vi "Average_array.vi"(1 "Input Array":dbl[](array[numeric]), 2 "Average over..":dbl) -> (0 "Output Array":dbl[](array[numeric]))   [LabVIEW 2016]
panel:
  out "Waveform Graph":dbl[](graph)
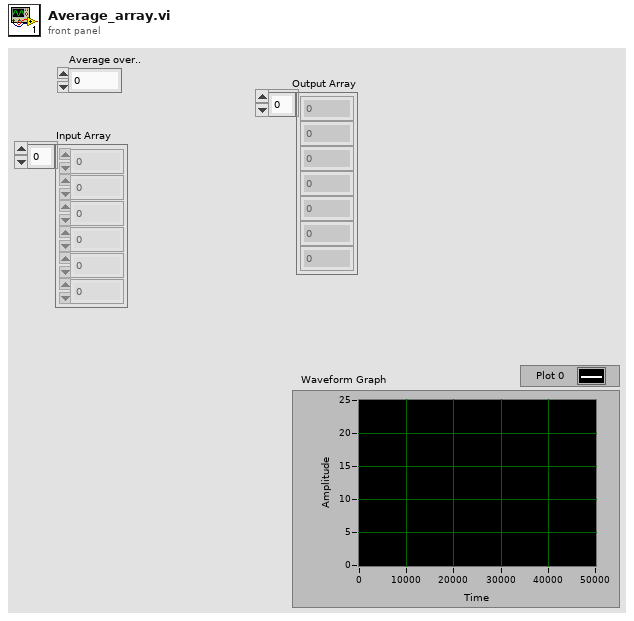
[diagram p1: front panel]
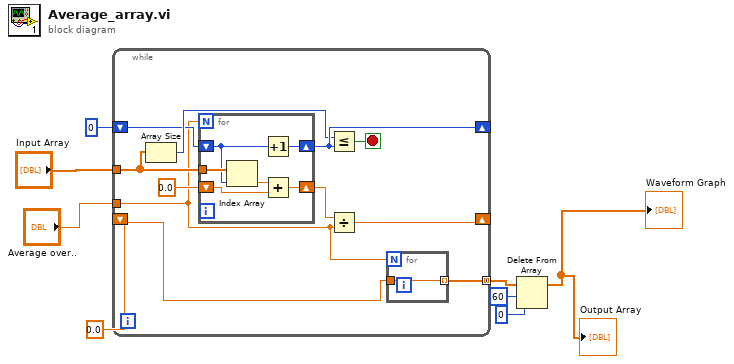
[diagram p0: block diagram]
diagram:
  n1 = while {
    tunnel: "Average over.." -> [w10]
    tunnel: "Input Array" -> [w16]
    shift-right: [w15] -> _
    shift-left: 0 -> [w13]
    shift-right: [w12] -> _
    shift-left: 0.0 -> [w9]
    tunnel: [w11] -> w4 mode=concatenating
    stop <- w19 stop-if-true
    n2 = Array Size(array=w16) -> (size(s)=w14:i32)
    n3 = for {
      N: w10 -> [_]
      tunnel: w16 -> [w26]
      shift-right: [w25] -> w18
      shift-left: 0.0 -> [w23]
      shift-right: [w22] -> w15
      shift-left: w13 -> [w21]
      n4 = Index Array(array=w26, index=w21) -> (element=w24:dbl)
      n5 = Increment(x=w21) -> (x+1=w22:i32)
      n6 = Add(x=w24, y=w23) -> (x+y=w25:dbl)
    }
    n7 = Less Or Equal?(x=w14, y=w15) -> (x <= y?=w19:bool)
    n8 = Divide(x=w18, y=w10) -> (x/y=w12:dbl)
    n9 = for {
      N: w10 -> [_]
      tunnel: w9 -> [w20]
      tunnel: [w20] -> w11 mode=indexing
    }
  }
  n10 = Delete From Array(array=w4, length=60, index=0) -> (array with subset deleted=→"Output Array" →"Waveform Graph":dbl[])  [unwired: 1 out]
